vi "Get Impulse Data as Reference.vi"(10 "Channel":i32, 11 "Reference in":T1) -> (2 "data value reference":refnum<data-value>, 3 "Reference out":T1)   [LabVIEW 2013, in "Impulse Data.lvclass"]
uses:
  Impulse Data.lvclass
  Instance handle.ctl
  Impulse Data.lvclass/Impulse Data.ctl
panel:
  out "error out":errorcluster
  in  "error in (no error)":errorcluster
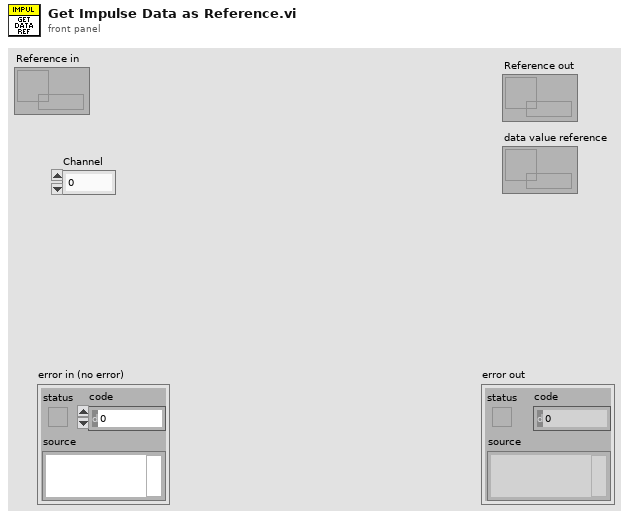
[diagram p1: front panel]
types:
  T1 = typedef "Impulse Data.lvclass/Instance handle.ctl" = refnum<data-value>
  T2 = typedef "TD_Impulse Planes.ctl" = enum16{"Other", "Yaw", "Pitch", "Roll", "LARP", "RALP"}
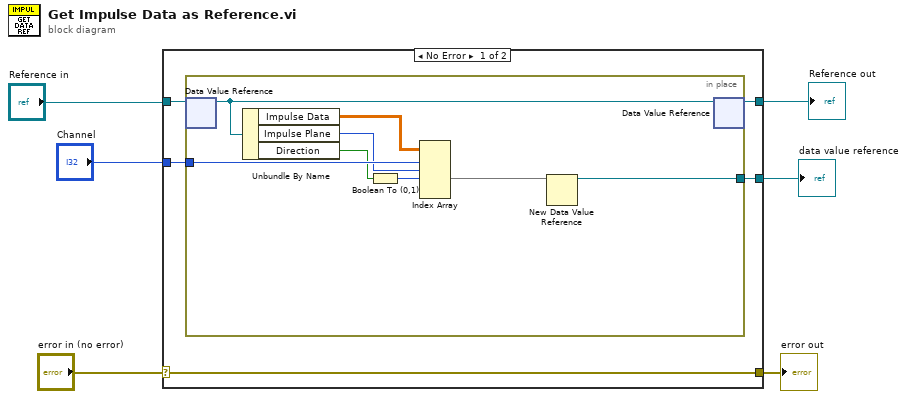
[diagram p0: block diagram]
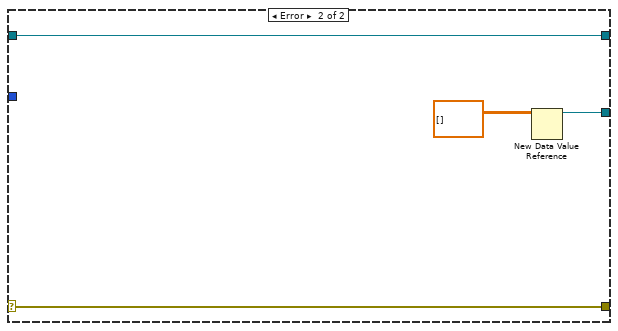
[diagram p2: hidden frame]
diagram:
  n1 = case shown="No Error" "error in (no error)" {
    selector: "error in (no error)" -> [w11 w23]
    tunnel: [w11 w23] -> w5
    tunnel: [w9 w22] -> w4
    tunnel: "Reference in" -> [w10 w22]
    tunnel: "Channel" -> [w8 _]
    tunnel: [w7 w20] -> w1
    frame No Error {
      n2 = in-place {
        in-place-border: w8 -> [w18]
        in-place-border: [w15] -> w7
        n3 = in-place-dvr #1(w10) -> (w17:refnum<class "Impulse Data.lvclass">)  [unwired: 1 out]
        n4 = Unbundle By Name(w17) -> ("Impulse Data"=w19:dbl[][][][][], "Impulse Plane"=w13:T2, "Direction"=w14:bool)
        n5 = Boolean To (0,1)(Boolean=w14) -> (0, 1=w12:i16)
        n6 = Index Array(array=w19, index (dim 0)=w18, index (dim 1)=w13, index (dim 2)=w12) -> (element=w16:dbl[][])  [unwired: 2 in]
        n7 = New Data Value Reference(data value=w16) -> (data value reference=w15:refnum<data-value>)  [unwired: 1 in, 1 out]
        n8 = in-place-dvr #1(w17) -> (w9:T1)  [unwired: 1 out]
      }
    }
    frame Error {
      n9 = New Data Value Reference(data value=dbl[][] [] ("subarray")) -> (data value reference=w20:refnum<data-value>)  [unwired: 1 in, 1 out]
    }
  }
  "error out" <- w5
  "Reference out" <- w4
  "data value reference" <- w1
